vi "CCWorklistSCU.vi"(6 "TimeCluster":T1, 7 "remotePort":i32=1234, 8 "error in (no error)":errorcluster, 9 "remoteHost":string="localhost", 10 "remoteAE":string="OFFIS", 11 "clientAETitle":string="PseudoSCU") -> (0 "error out":errorcluster, 1 "patientsRetrieved":i32, 2 "Worklist":string[][](array[string]), 3 "DicomTags":string[](array[string]), 5 "Find":refnum<k24>)   [LabVIEW 2013, in "main.lvlib" / "ClearCanvasLibrary.lvlib"]
uses:
  ClearCanvasLibrary.lvlib
  C:/Users/Simon/SkyDrive/LabView/2013/DM2020/DICOM/ClearCanvasNewBuild/ClearCanvas.Dicom.dll
  ClearCanvasNewBuild/ClearCanvas.Dicom.dll
  main.lvlib
  Controls/Enum Variables.ctl
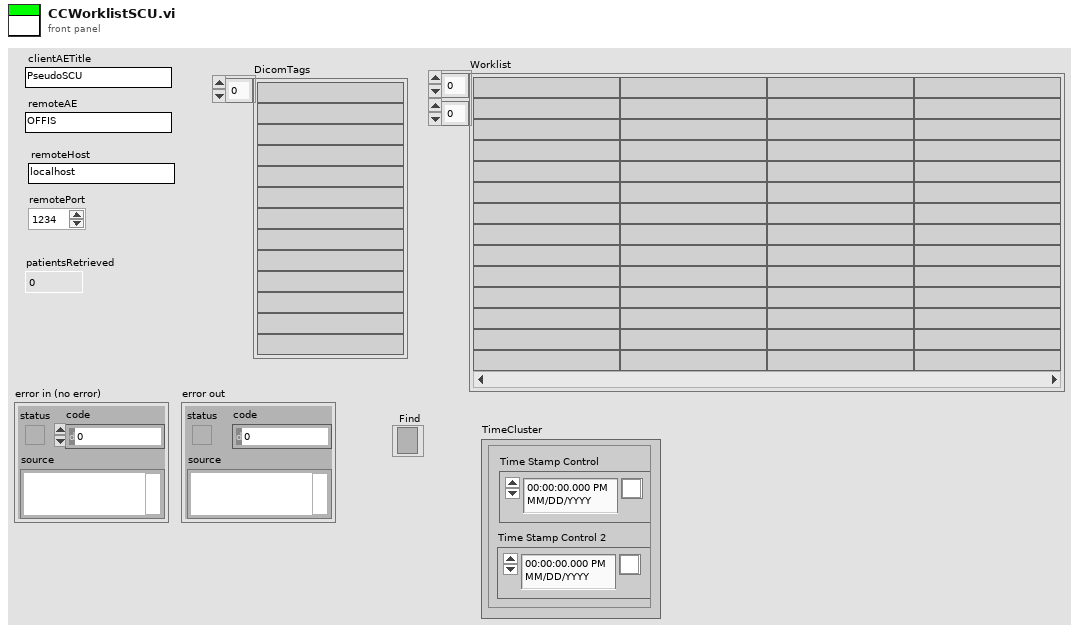
[diagram p1: front panel]
types:
  T1 = cluster{"Time Stamp Control":timestamp, "Time Stamp Control 2":timestamp}
  T2 = typedef "main.lvlib/Enum Variables.ctl" = enum16{"SetAcqFilter", "GetAcqFilter", "Set Filter", "Get Filter", "Set Height", "Get Height", "Set Blue Pressure", "Get Blue Pressure", "Set Red Pressure", "Get Red Pressure", "Init", "Reset Pressure", "Set Red Cursors", "Get Red Cursors", "Set Blue Cursors", "Get Blue Cursors", "Set Language", "Get Language", "Set Active Graphs", "Get ActiveGraphs", "Set Method", "Get Method", "Set Encryption", "Get Encryption", "Set ExcelVersion", "Get ExcelVersion", "Set DICOM Avail", "Get DICOM Avail", "Set DICOM Encode", "Get DICOM Encode", "Set JournalExport", "Get JournalExport", "Set Sequence", "Get Sequence", "Set DAQ Connected", "Get DAQ Connected", "Set Current Graph", "Get Current Graph", "Set General Settings", "Get Hyphenation", "Set Arm Calc Method", "Get Arm Calc Method", "Set Dicom Tags", "Get Dicom Tags", "Set BT Serial", "Get BT Serial", "Set BT Accepted Serials", "Get BT Accepted Serials", "Get BT License", "Set BT License"}
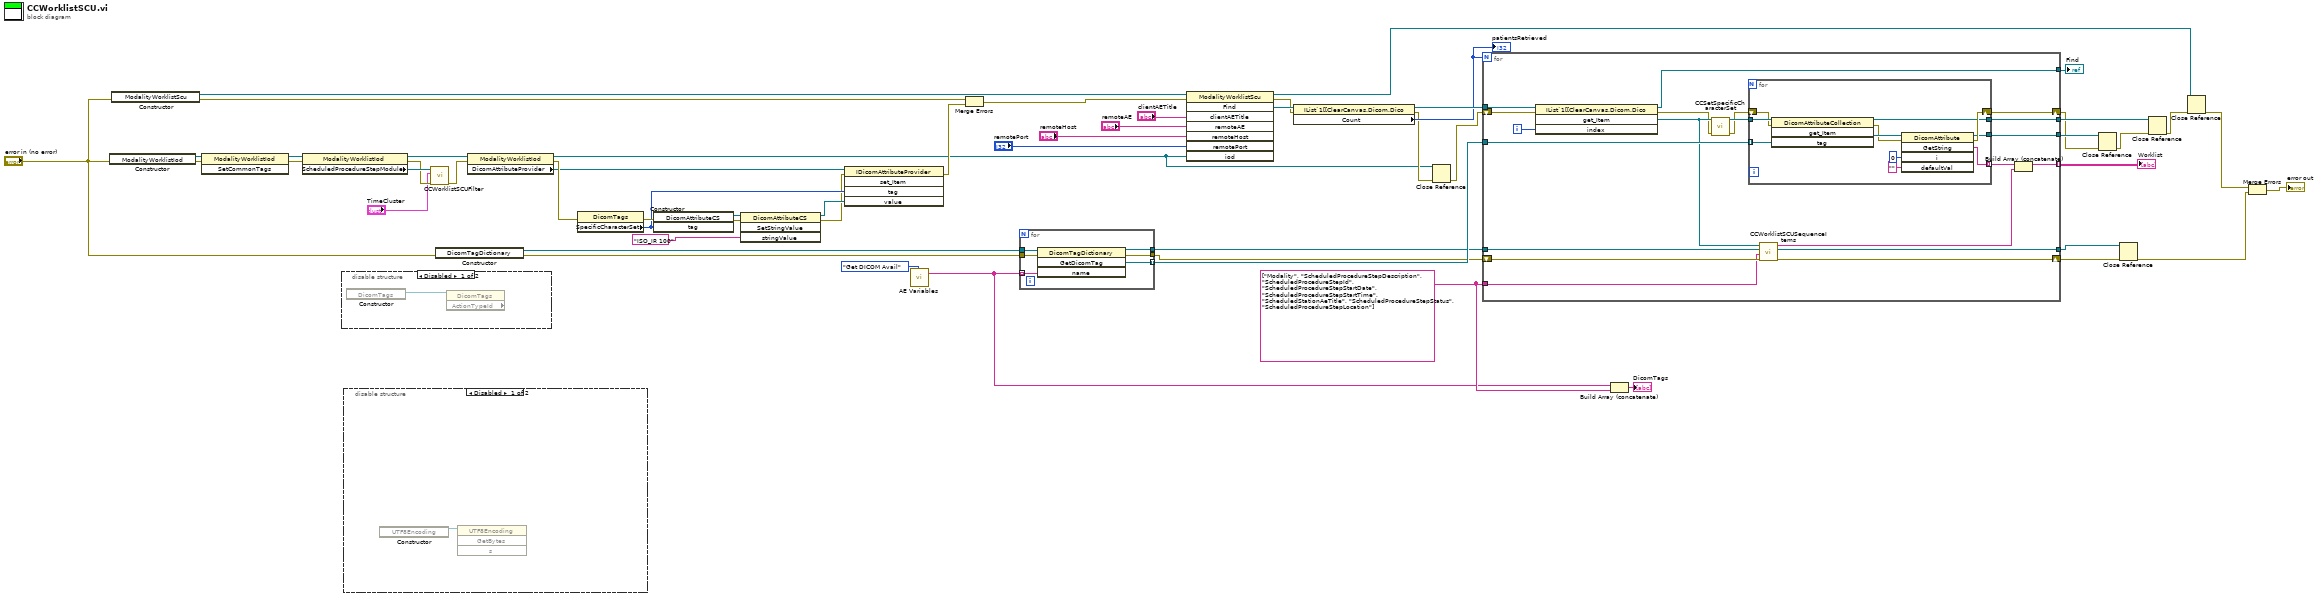
[diagram p0: block diagram]
diagram:
  w37 = string[] ["Modality", "ScheduledProcedureStepDescription", "ScheduledProcedureStepId", "ScheduledProcedureStepStartDate", "ScheduledProcedureStepStartTime", "ScheduledStationAeTitle", "ScheduledProcedureStepStatus", "ScheduledProcedureStepLocation"]
  n1 = constructor class="ModalityWorklistIod"(error in="error in (no error)") -> (reference out=w55:refnum<k24>, error out=w50:errorcluster)  [unwired: 2 in, 1 out]
  n2 = constructor class="ModalityWorklistScu"(error in="error in (no error)") -> (reference out=w56:refnum<k24>, error out=w20:errorcluster)  [unwired: 2 in, 1 out]
  n3 = invoke class="ModalityWorklistIod" method="SetCommonTags"(reference=w55, error in=w50) -> (reference out=w25:refnum<k24>, error out=w23:errorcluster)  [unwired: 1 in, 1 out]
  n4 = property class="ModalityWorklistIod"(reference=w25, error in=w23) -> (reference out=w13:refnum<k24>, error out=w22:errorcluster, "ScheduledProcedureStepModule"=w24:refnum<k24>)
  n5 = disable-structure shown="Disabled" {
    frame Disabled {
      n6 = constructor class="DicomTags"() -> (reference out=w57:refnum<k24>)  [unwired: 3 in, 2 out]
      n7 = property class="DicomTags" props=["ActionTypeId"](reference=w57) -> ()  [unwired: 1 in, 3 out]
    }
    frame Enabled {
    }
  }
  n8 = disable-structure shown="Disabled" {
    frame Disabled {
      n9 = constructor class="UTF8Encoding"() -> (reference out=w58:refnum<k24>)  [unwired: 3 in, 2 out]
      n10 = invoke class="UTF8Encoding" method="GetBytes"(reference=w58) -> ()  [unwired: 3 in, 4 out]
    }
    frame Enabled {
    }
  }
  n11 = call "CCWorklistSCUFilter.vi"("error in (no error)"=w22, "TimeCluster"="TimeCluster", ".NET Refnum in"=w24) -> ("error out"=w5:errorcluster)  [unwired: 8 in]
  n12 = constructor class="DicomTagDictionary"(error in="error in (no error)") -> (reference out=w34:refnum<k24>, error out=w49:errorcluster)  [unwired: 2 in, 1 out]
  n13 = property class="ModalityWorklistIod"(reference=w13, error in=w5) -> (reference out=w2:refnum<k24>, error out=w4:errorcluster, "DicomAttributeProvider"=w1:refnum<k24>)
  n14 = property class="DicomTags"(error in=w4) -> (error out=w9:errorcluster, "SpecificCharacterSet"=w8:u32)  [unwired: 1 in, 1 out]
  n15 = constructor class="DicomAttributeCS"(error in=w9, "tag"=w8) -> (reference out=w10:refnum<k24>, error out=w11:errorcluster)  [unwired: 2 in, 2 out]
  n16 = invoke class="DicomAttributeCS" method="SetStringValue"(reference=w10, error in=w11, "stringValue"="ISO_IR 100") -> (reference out=w7:refnum<k24>, error out=w6:errorcluster)  [unwired: 1 in, 2 out]
  n17 = invoke class="IDicomAttributeProvider" method="set_Item"(reference=w1, error in=w6, "tag"=w8, "value"=w7) -> (error out=w3:errorcluster)  [unwired: 1 in, 4 out]
  n18 = call "AE Variables.vi"("Action"=Enum_Variables."Get DICOM Avail") -> ("stringArray"=w14:string[])  [unwired: 11 in, 7 out]
  n19 = Merge Errors(w20, w3) -> (w19:errorcluster)
  n20 = for {
    tunnel: w34 -> [w64]
    tunnel: w49 -> [w63]
    tunnel: w14 -> [w62] mode=indexing
    tunnel: [w61] -> w46 mode=indexing
    tunnel: [w60] -> w26
    tunnel: [w59] -> w45
    n21 = invoke class="DicomTagDictionary" method="GetDicomTag"(reference=w64, error in=w63, "name"=w62) -> (reference out=w60:refnum<k24>, error out=w59:errorcluster, "GetDicomTag"=w61:refnum<k24>)  [unwired: 1 in, 1 out]
  }
  n22 = invoke class="ModalityWorklistScu" method="Find"(reference=w56, error in=w19, "clientAETitle"="clientAETitle", "remoteAE"="remoteAE", "remoteHost"="remoteHost", "remotePort"="remotePort", "iod"=w2) -> (reference out=w33:refnum<k24>, error out=w18:errorcluster, "Find"=w48:refnum<k24>)  [unwired: 1 in, 5 out]
  n23 = property class="IList`1[[ClearCanvas.Dicom.Dico"(reference=w48, error in=w18) -> (reference out=w47:refnum<k24>, error out=w17:errorcluster, "Count"=w44:i32)
  "patientsRetrieved" <- w44
  n24 = Close Reference(reference=w2, error in (no error)=w17) -> (error out=w16:errorcluster)
  n25 = for {
    N: w44 -> [_]
    tunnel: w47 -> [w74]
    tunnel: w46 -> [w82]
    tunnel: [w76] -> w35 mode=indexing
    shift-right: [w83] -> w29
    shift-left: w16 -> [w73]
    tunnel: w26 -> [w72]
    tunnel: w37 -> [w79]
    shift-right: [w78] -> w42
    shift-left: w45 -> [w80]
    tunnel: [w72] -> w43
    tunnel: [w71] -> w32
    tunnel: [w70] -> w30
    tunnel: [w69] -> w31
    i -> [w81]
    n26 = invoke class="IList`1[[ClearCanvas.Dicom.Dico" method="get_Item"(reference=w74, error in=w73, "index"=w81) -> (reference out=w71:refnum<k24>, error out=w66:errorcluster, "get_Item"=w68:refnum<k24>)  [unwired: 1 in, 1 out]
    n27 = call "CCSetSpecificCharacterSet.vi"("error in (no error)"=w66, ".NET Refnum in"=w68) -> ("error out"=w65:errorcluster, ".NET Refnum out"=w67:refnum<k24>)  [unwired: 8 in]
    n28 = for {
      tunnel: [w84] -> w77 mode=indexing
      shift-right: [w90] -> w83
      shift-left: w65 -> [w87]
      tunnel: w82 -> [w89] mode=indexing
      tunnel: w67 -> [w88]
      tunnel: [w86] -> w70
      tunnel: [w85] -> w69
      n29 = invoke class="DicomAttributeCollection" method="get_Item"(reference=w88, error in=w87, "tag"=w89) -> (reference out=w85:refnum<k24>, error out=w91:errorcluster, "get_Item"=w94:refnum<k24>)  [unwired: 1 in, 1 out]
      n30 = invoke class="DicomAttribute" method="GetString"(reference=w94, error in=w91, "i"=0, "defaultVal"="") -> (reference out=w86:refnum<k24>, error out=w90:errorcluster, "GetString"=w84:string)  [unwired: 1 in, 2 out]
    }
    n31 = call "CCWorklistSCUSequenceItems.vi"("error in (no error)"=w80, "Array in"=w79, "new reference"=w72, ".NET Refnum in"=w68) -> ("error out"=w78:errorcluster, "Array out"=w75:string[])  [unwired: 6 in]
    n32 = Build Array (concatenate)(w77, w75) -> (w76:string[])
  }
  "Worklist" <- w35
  "Find" <- w32
  n33 = Build Array (concatenate)(w14, w37) -> (→"DicomTags":string[])
  n34 = Close Reference(reference=w30, error in (no error)=w29) -> (error out=w28:errorcluster)
  n35 = Close Reference(reference=w43, error in (no error)=w42) -> (error out=w40:errorcluster)
  n36 = Close Reference(reference=w31, error in (no error)=w28) -> (error out=w27:errorcluster)
  n37 = Close Reference(reference=w33, error in (no error)=w27) -> (error out=w41:errorcluster)
  n38 = Merge Errors(w41, w40) -> (→"error out":errorcluster)
